vi "Read Analog Input Values.vi"(8 "error in":errorcluster, 9 "Timeout / s":dbl=10.0 format="%0.2f", 10 "AI ULx Task":refnum<k24>, 11 "BNT_ULx-MCSV-AIAvg in":refnum<class "BNT_ULx-MCSV-AIAvg.lvclass">) -> (0 "error out":errorcluster, 1 "AI Data":dbl[](array[numeric]), 3 "BNT_ULx-MCSV-AIAvg out":refnum<class "BNT_ULx-MCSV-AIAvg.lvclass">)   [LabVIEW 2020, in "BNT_ULx.lvlib" / "BNT_ULx-MCSV-AIAvg.lvclass"]
doc: "Read analog input.\n\n<b>Default Implementation:</b> Analog Input\n\nThis dynamic dispatch VI can be overritten by derived classes to implement other analog input readings."
uses:
  BNT_ULx-MCSV-AIAvg.lvclass
  BNT_ULx-MCSV-AIAvg.lvclass/BNT_ULx-MCSV-AIAvg.ctl
  <vilib>/Analysis/NI_AALBase.lvlib
  CSPP_Core/Libraries/Utilities/CSPP_Utilities.lvlib
  <vilib>/ULx/Read.llb/ULx Read (Analog 2D DBL NChan NSamp).vi
  <vilib>/Analysis/baseanly.llb/Mean (DBL).vi
  C:/Program Files (x86)/National Instruments/LabVIEW 2020/vi.lib/ULx/ULx_LV.dll
  Program Files (x86)/National Instruments/LabVIEW 2020/vi.lib/ULx/ULx_LV.dll
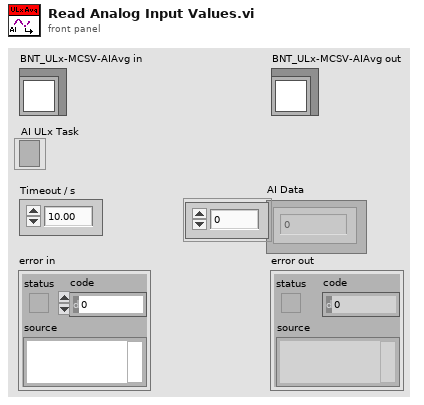
[diagram p1: front panel]
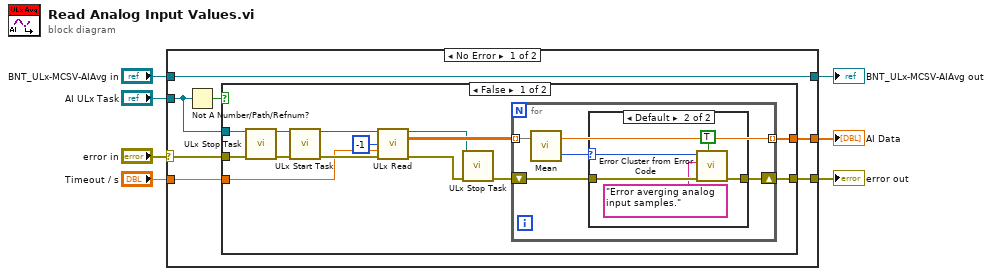
[diagram p0: block diagram]
diagram:
  n1 = case shown="No Error" "error in" {
    selector: "error in" -> [w13 w42]
    tunnel: [w12 w42] -> w2
    tunnel: [w8 w41] -> w4
    tunnel: "BNT_ULx-MCSV-AIAvg in" -> [w8 w41]
    tunnel: "Timeout / s" -> [w14 _]
    tunnel: [w11 _] -> w3
    tunnel: "AI ULx Task" -> [w9 _]
    frame No Error {
      n2 = Not A Number/Path/Refnum?(number/path/refnum=w9) -> (NaN/Path/Refnum?=w10:bool)
      n3 = case shown="False" w10 {
        tunnel: w14 -> [w18 _]
        tunnel: w13 -> [w20 w40]
        tunnel: [w27 w40] -> w12
        tunnel: [w28 _] -> w11
        tunnel: w9 -> [w25 _]
        frame False {
          n4 = call <vilib>:"ULx Stop Task.vi"("error in"=w20, "task in"=w25) -> ("error out"=w21:errorcluster, "task out"=w24:refnum<k24>)  [unwired: 8 in]
          n5 = call <vilib>:"ULx Start Task.vi"("task in"=w24, "error in"=w21) -> ("task out"=w23:refnum<k24>, "error out"=w22:errorcluster)  [unwired: 12 in]
          n6 = call-poly <vilib>:"ULx Read.vi"("task in"=w23, "number of samples per channel"=-1, "timeout"=w18, "error in"=w22) -> ("task out"=w19:refnum<k24>, "data"=w26:dbl[][], "error out"=w16:errorcluster)  [unwired: 9 in]
          n7 = call <vilib>:"ULx Stop Task.vi"("error in"=w16, "task in"=w19) -> ("error out"=w15:errorcluster)  [unwired: 8 in, 1 out]
          n8 = for {
            tunnel: w26 -> [w33] mode=indexing
            tunnel: [w32] -> w28 mode=indexing
            shift-right: [w30] -> w27
            shift-left: w15 -> [w29]
            n9 = call-poly <vilib>:"Mean.vi"("X"=w33) -> ("mean"=w32:dbl, "error"=w31:i32)
            n10 = case shown="Default" w31 {
              selector: w31 -> [_ w39]
              tunnel: [w34 w38] -> w30
              tunnel: w29 -> [w34 w37]
              frame 0 {
              }
              frame Default {
                n11 = call "Error Cluster from Error Code.vi"("show call chain? (False)"=TRUE, "Error In"=w37, "Error Message (\"\")"="Error averging analog input samples." ("error message (\"\")"), "Error Code (0)"=w39) -> ("Error Out"=w38:errorcluster)  [unwired: 7 in]
              }
            }
          }
        }
        frame True {
        }
      }
    }
    frame Error {
    }
  }
  "error out" <- w2
  "BNT_ULx-MCSV-AIAvg out" <- w4
  "AI Data" <- w3
